vi "DAQ Matrix Size (SubVI).vi"(6 "LC Array":dbl[](array[numeric]), 8 "System Signals":dbl[](array[numeric]), 9 "LS Array":dbl[](array[numeric]), 10 "TC Array":dbl[](array[numeric]), 11 "PT Array":dbl[](array[numeric])) -> (3 "Output Matrix":dbl[][](array[numeric]))   [LabVIEW 2020]
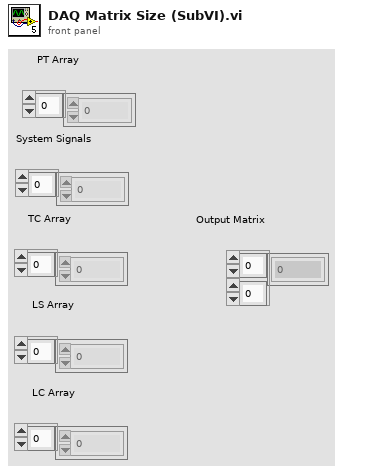
[diagram p1: front panel]
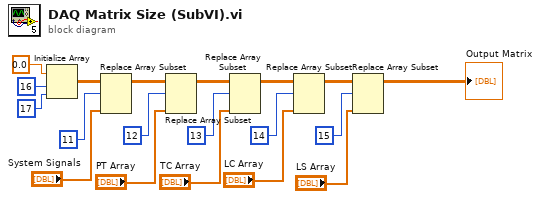
[diagram p0: block diagram]
diagram:
  n1 = Initialize Array(0.0 ("element"), 16 ("dimension size"), 17 ("dimension size")) -> (w5:dbl[][])
  n2 = Replace Array Subset(array=w5, new element="System Signals", index (row)=11) -> (w4:dbl[][])  [unwired: 1 in]
  n3 = Replace Array Subset(array=w4, new element="PT Array", index (row)=12) -> (w16:dbl[][])  [unwired: 1 in]
  n4 = Replace Array Subset(array=w16, new element="TC Array", index (row)=13) -> (w17:dbl[][])  [unwired: 1 in]
  n5 = Replace Array Subset(array=w17, new element="LC Array", index (row)=14) -> (w18:dbl[][])  [unwired: 1 in]
  n6 = Replace Array Subset(array=w18, new element="LS Array", index (row)=15) -> (→"Output Matrix":dbl[][])  [unwired: 1 in]
